vi "Atto DRY Interface get40K Stage Temperature.vi"(8 "error in (no error)":errorcluster, 11 "_40KStageTemperatureK":sgl) -> (0 "error out":errorcluster, 2 "function return":i32, 3 "_40KStageTemperatureK out":sgl)   [LabVIEW 2016, in "attoDRYLib.lvlib"]
doc: "int32_t __cdecl AttoDRY_Interface_get40KStageTemperature(\n float *_40KStageTemperatureK);"
uses:
  <userlib>/attoDRYLib/attoDRYLib.lvlib
  <userlib>/attoDRYLib/attoDRYLib.dll
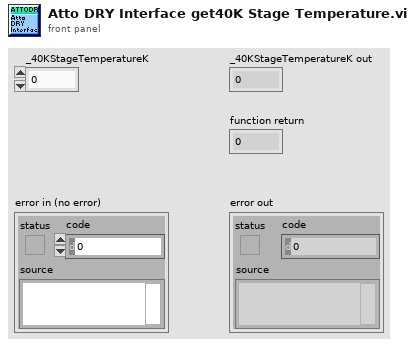
[diagram p1: front panel]
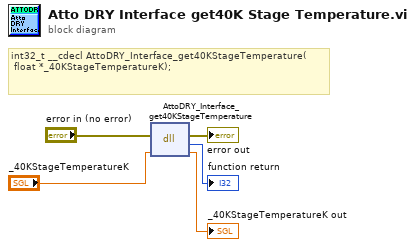
[diagram p0: block diagram]
diagram:
  # "int32_t __cdecl AttoDRY_Interface_get40KStageTemperature(\n\tfloat *_40KStageTemperatureK);"
  n1 = dll-call lib="C:/Program Files (x86)/National Instruments/LabVIEW 2016/user.lib/attoDRYLib/attoDRYLib.*" fn="AttoDRY_Interface_get40KStageTemperature"(error in="error in (no error)", "_40KStageTemperatureK"="_40KStageTemperatureK") -> (error out=→"error out":errorcluster, →"function return":i32, "_40KStageTemperatureK"=→"_40KStageTemperatureK out":sgl)  [unwired: 2 in, 1 out]
